vi "Loop.vi"() -> ()   [LabVIEW 2012]
panel:
  out "?":dbl(graph)
  in  "stop":bool
  in  "Millisecond Display":dbl(slide) scale=0.0..10.0
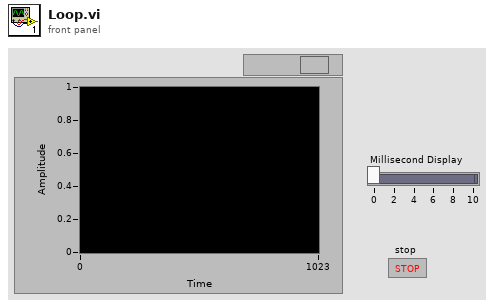
[diagram p1: front panel]
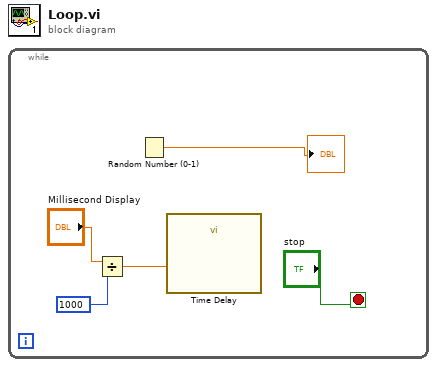
[diagram p0: block diagram]
diagram:
  n1 = while {
    stop <- "stop" stop-if-true
    n2 = Divide(x="Millisecond Display", y=1000) -> (x/y=w1:dbl)
    n3 = Random Number (0-1)() -> (number: 0 to 1=→"?":dbl)
    n4 = call "Time Delay"("Delay Time (s)"=w1) -> ()  [unwired: 10 in, 1 out]
  }
